vi "Parse Fix Mode.vi"(10 "Mode Index":i32, 11 "Fields In":string[](array[string])) -> (2 "Fix Mode":T1, 3 "Fields":string[](array[string]))   [LabVIEW 2020, in "nmea.lvlib" / "nmea.lvclass"]
uses:
  nmea.lvclass
  Fix Mode.ctl
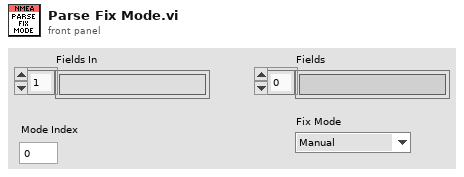
[diagram p1: front panel]
types:
  T1 = typedef "nmea.lvlib/nmea.lvclass/Fix Mode.ctl" = enum16{"Manual", "Auto 2/3D"}
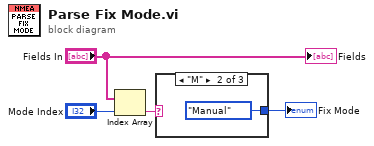
[diagram p0: block diagram]
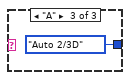
[diagram p3: hidden frame]
diagram:
  n1 = Index Array(array="Fields In", index="Mode Index") -> (element=w2:string)
  n2 = case shown="\"M\"" w2 {
    tunnel: [_ Fix_Mode."Manual" ("Fix Mode") Fix_Mode."Auto 2/3D" ("Fix Mode")] -> w1
    frame Default {
    }
    frame "M" {
    }
    frame "A" {
    }
  }
  "Fix Mode" <- w1
  "Fields" <- "Fields In"
